vi "startSensors.vi"(2 "MXP Port":enum16{"A", "B"}(ring), 3 "CAN ID":u32 format="%x") -> (0 "IMU Config Out":T1, 1 "SPI Configs Out":T3)   [LabVIEW 2019]
uses:
  SPI/SPI Config.ctl
  MPU 9250/IMU Config.ctl
panel:
  in  "SPI Configs Reference":T3
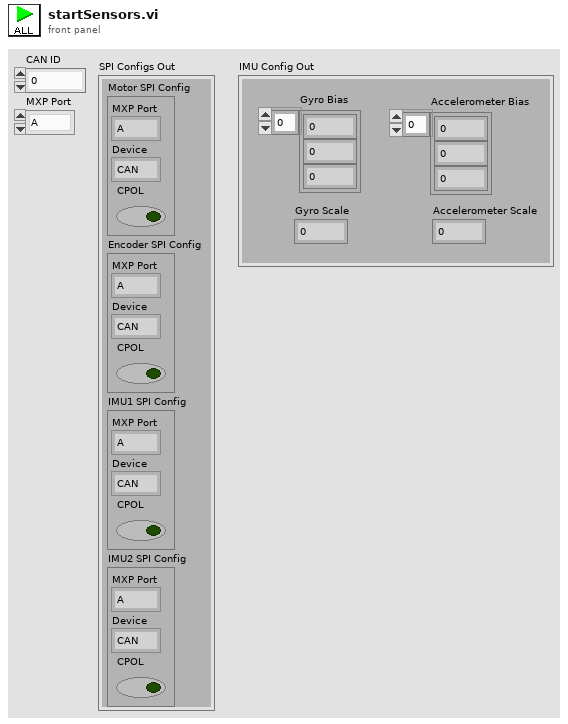
[diagram p1: front panel]
types:
  T1 = typedef "IMU Config.ctl" = cluster{"Accelerometer Bias":i16[], "Accelerometer Scale":i16, "Gyro Bias":i16[], "Gyro Scale":i16}
  T2 = typedef "SPI Config.ctl" = cluster{"MXP Port":enum16{"A", "B"}, "Device":enum16{"CAN", "ENC", "IMU1", "IMU2"}, "CPOL":bool}
  T3 = cluster{"Motor SPI Config":T2, "Encoder SPI Config":T2, "IMU1 SPI Config":T2, "IMU2 SPI Config":T2}
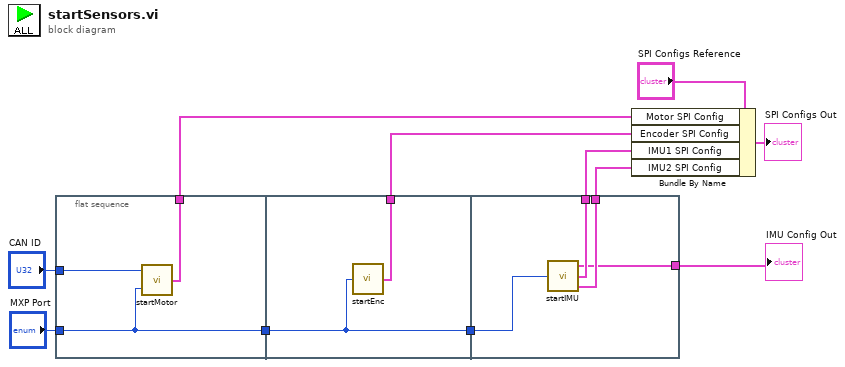
[diagram p0: block diagram]
diagram:
  n1 = flat-sequence {
    tunnel: "CAN ID" -> [w14]
    tunnel: "MXP Port" -> [w13]
    tunnel: [w13] -> w9
    tunnel: [w12] -> w7
    tunnel: w9 -> [w16]
    tunnel: [w16] -> w8
    tunnel: [w15] -> w6
    tunnel: w8 -> [w20]
    tunnel: [w19] -> w5
    tunnel: [w18] -> w4
    tunnel: [w17] -> w1
    frame #0 {
      n2 = call "startMotor.vi"("MXP Port"=w13, "ID"=w14) -> ("SPI Config Out"=w12:T2)
    }
    frame #1 {
      n3 = call "startEnc.vi"("MXP Port"=w16) -> ("SPI Config Out"=w15:T2)
    }
    frame #2 {
      n4 = call "startIMU.vi"("MXP Port"=w20) -> ("IMU Config Out"=w17:T1, "IMU1 SPI Config"=w19:T2, "IMU2 SPI Config"=w18:T2)
    }
  }
  n5 = Bundle By Name(cluster="SPI Configs Reference", "Motor SPI Config"=w7, "Encoder SPI Config"=w6, "IMU1 SPI Config"=w5, "IMU2 SPI Config"=w4) -> (→"SPI Configs Out":T3)
  "IMU Config Out" <- w1
